vi "Scalar JSON text to Variant.vi"(6 "Type":T1, 8 "error in (no error)":errorcluster, 9 "Variant (Data Type)":variant, 10 "Offset":i32, 11 "JSON":string) -> (0 "error out":errorcluster, 1 "Variant out":variant)   [LabVIEW 2017, in "JSONtext.lvlib"]
uses:
  JSONtext.lvlib
  <vilib>/Utility/Data Type/Type Definitions/Data Type.ctl
  <vilib>/Utility/Data Type/Type Definitions/Refnum Type.ctl
  Advance past String.vi
  String Subset.vi
  support/Strip Quotes and Unescape.vi
  support/Get Number Text.vi
  NaN or null to Integer ERROR.vi
  Advance past Number.vi
  Parsing Error in converting to LabVIEW type.vi
  support/Unescape JSON string.vi
  <vilib>/JDP Science/JDP Science Common Utilities/Timestamp/Text to Timestamp.vi
  <vilib>/Utility/Data Type/NI_Data Type.lvlib
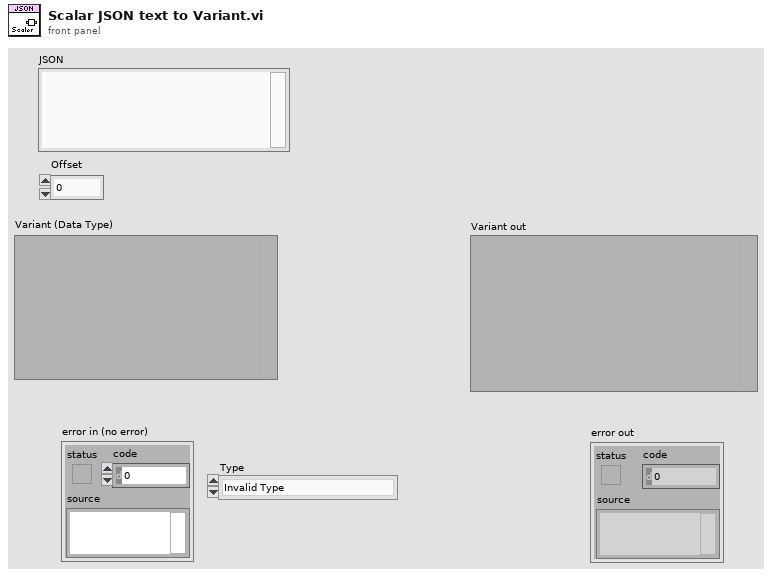
[diagram p1: front panel]
types:
  T1 = typedef "NI_Data Type.lvlib/Data Type.ctl" = enum8{"Invalid Type", "Void", "I8", "I16", "I32", "I64", "U8", "U16", "U32", "U64", "Single Float", "Double Float", "Extended Float", "Single Complex", "Double Complex", "Extended Complex", "Enum U8", "Enum U16", "Enum U32", "Enum U64", "Single Float With Unit", "Double Float With Unit", "Extended Float With Unit", "Single Complex with Unit", "Double Complex with Unit", "Extended Complex with Unit", "Boolean", "String", "Path", "Picture", "Tag", "Array", "Cluster", "Variant", "LV Variant", "Waveform", "Timestamp", "Digital Waveform", "Digital Data", "ExpressData", "Refnum", "External Data", "VI", "Poly VI", "LabVIEW Class Instance", "Fixed Point"}
  T2 = typedef "JSONtext.lvlib/Parsing State.ctl" = enum16{"Parser Error", "Object", "Array", "String", "Number/Other", "Leading Whitespace", "Object end", "Array end", "Value end"}
  T3 = typedef "NI_Data Type.lvlib/Refnum Type.ctl" = enum16{"NotARefnum", "UnknownRefnum", "Generic", "Datalog", "ByteStream", "Device", "Occurence", "TCPNetConnection", "Auto", "Menu", "Imaq", "Hardware", "DataSocket", "Visa", "IVI", "UDPNetConnection", "Notifier", "Queue", "Irda", "EventReg", "DotNet", "UserEvent", "Callback", "UNUSED_EMPTY_POSITION", "BlueToothNetConnection", "LVObjApp", "LVObjVI", "LVObjUnknown", "GenericClass", "UserDefinedRefnumTag", "DataValue", "RT FIFO", "TDMS File"}
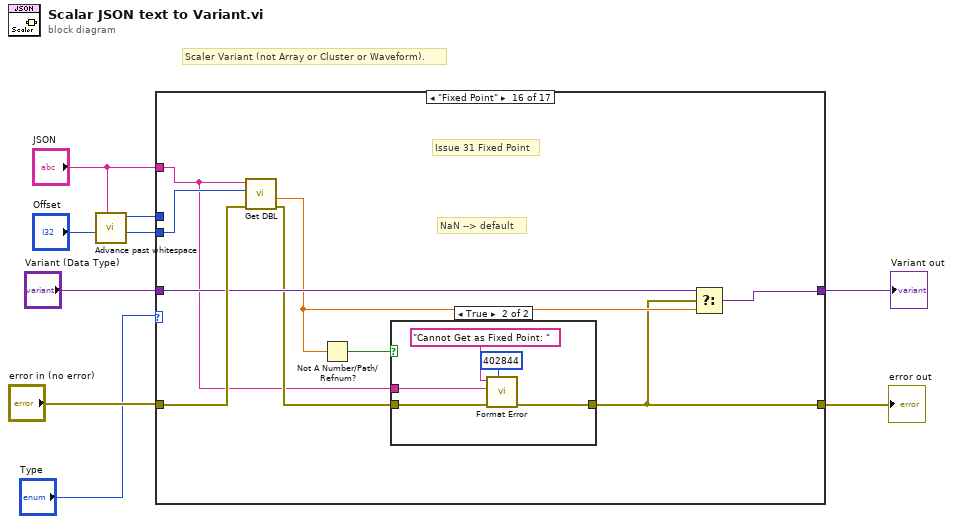
[diagram p0: block diagram]
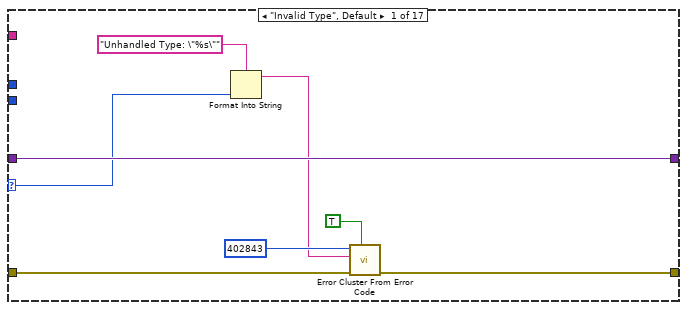
[diagram p2: hidden frame]
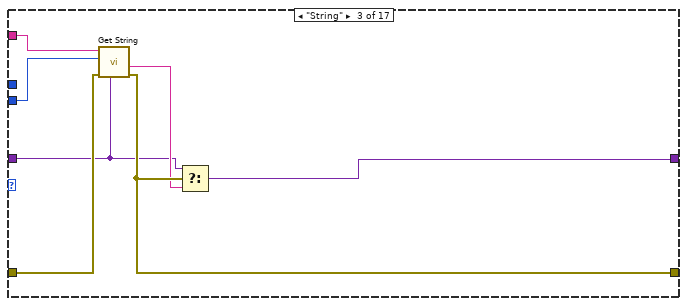
[diagram p4: hidden frame]
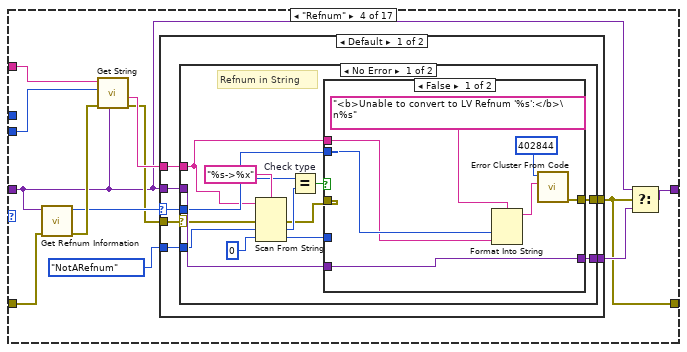
[diagram p5: hidden frame]
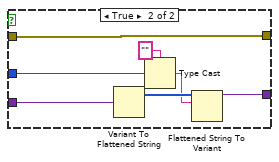
[diagram p6: hidden frame]
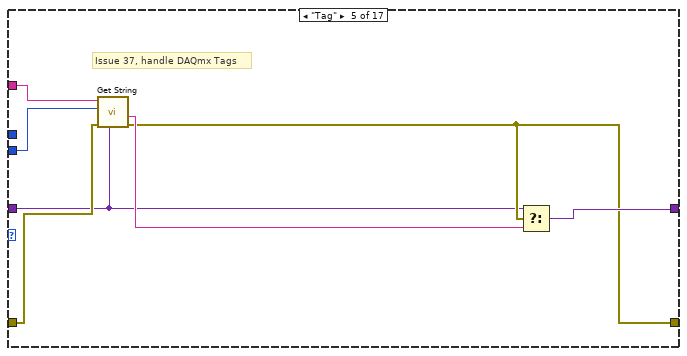
[diagram p9: hidden frame]
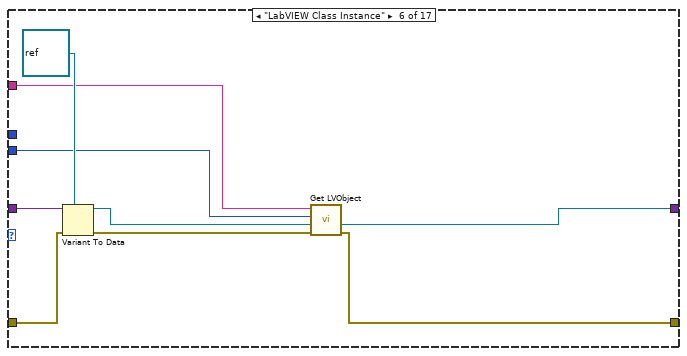
[diagram p10: hidden frame]
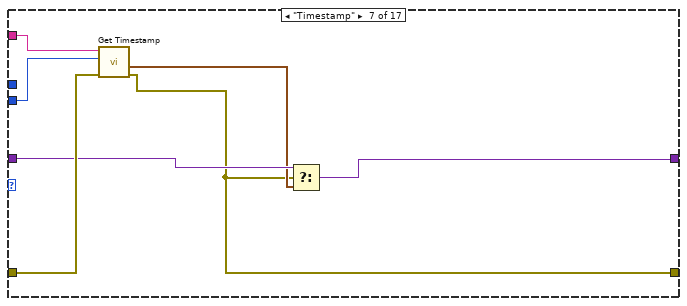
[diagram p11: hidden frame]
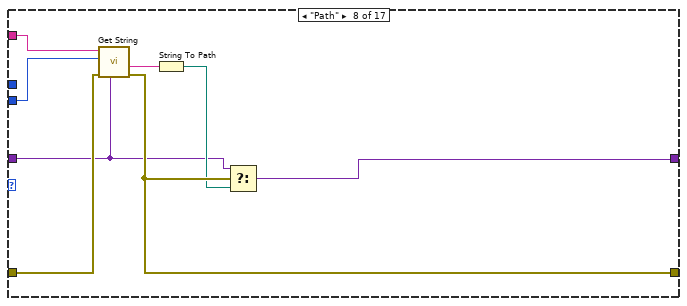
[diagram p12: hidden frame]
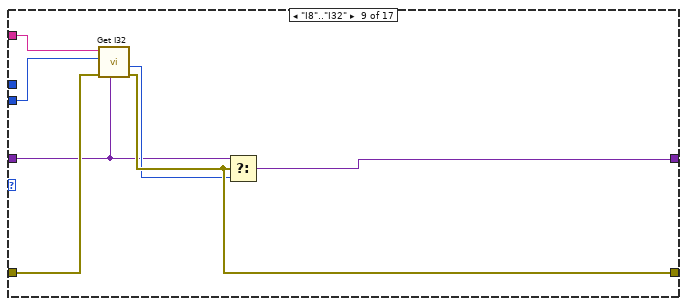
[diagram p13: hidden frame]
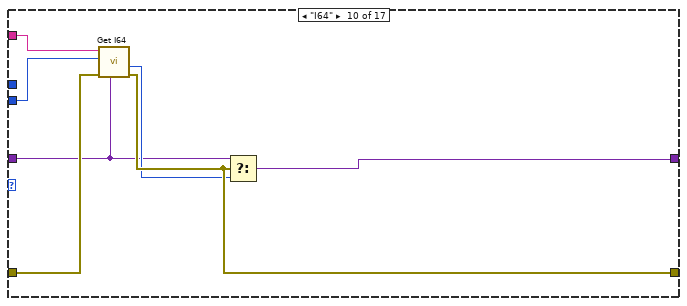
[diagram p14: hidden frame]
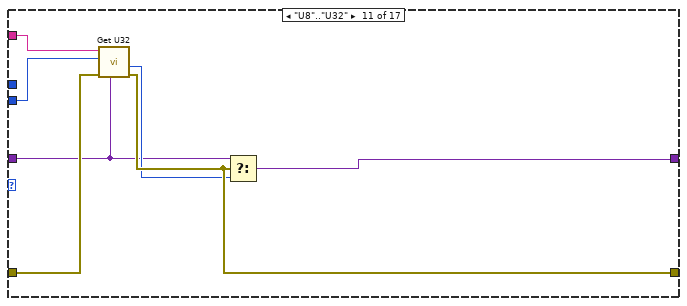
[diagram p15: hidden frame]
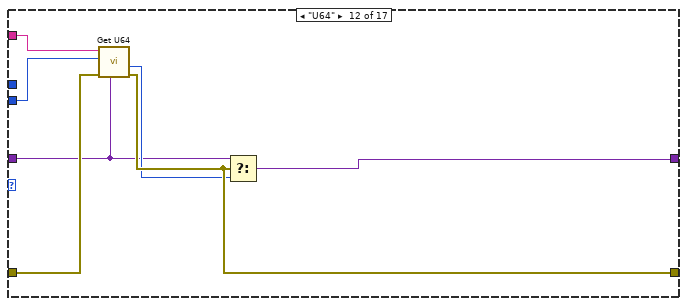
[diagram p16: hidden frame]
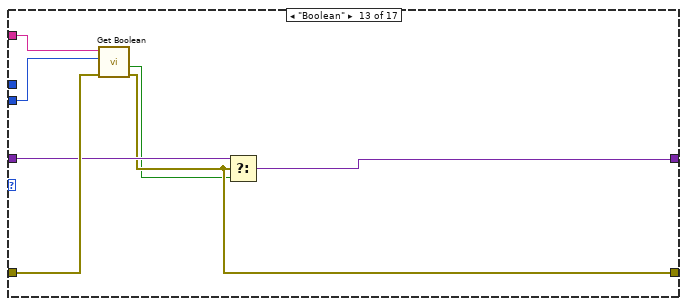
[diagram p17: hidden frame]
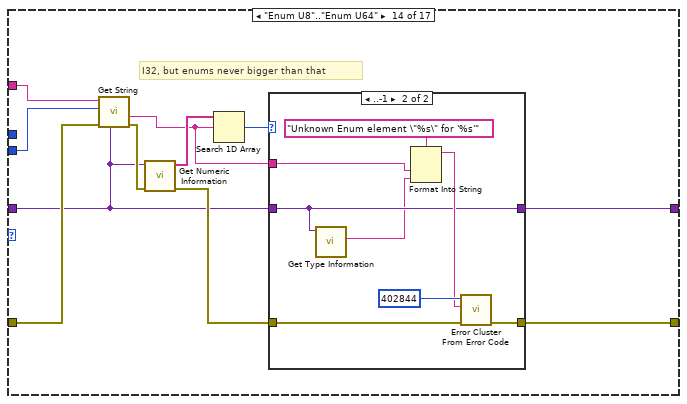
[diagram p18: hidden frame]
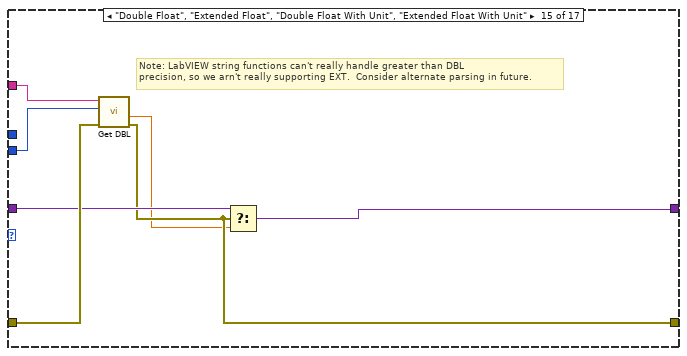
[diagram p20: hidden frame]
diagram:
  # "Scaler Variant (not Array or Cluster or Waveform)."
  n1 = call "Advance past whitespace.vi"("JSON"="JSON", "Offset"="Offset") -> ("Offset of first non-whitespace"=w5:i32, "Parser State"=w3:T2)  [unwired: 8 in]
  n2 = case shown="\"Fixed Point\"" "Type" {
    selector: "Type" -> [w12 _ _ _ _ _ _ _ _ _ _ _ _ _ _ _ _]
    tunnel: "Variant (Data Type)" -> [w16 w18 w20 w27 w76 w90 w95 w99 w107 w114 w121 w128 w139 w142 w167 w176 w189]
    tunnel: "JSON" -> [_ _ w25 w37 w81 w84 w97 w105 w109 w116 w123 w130 w136 w150 w164 w172 w186]
    tunnel: [w15 w19 w22 w29 w77 w89 w92 w102 w110 w117 w124 w131 w137 w146 w165 w170 w187] -> w8
    tunnel: "error in (no error)" -> [w17 w19 w24 w35 w79 w88 w96 w104 w112 w119 w126 w133 w140 w151 w168 w177 w190]
    tunnel: w5 -> [_ _ w26 w38 w82 w85 w98 w106 w113 w120 w127 w134 w141 w152 w169 w178 w191]
    tunnel: [w16 w18 w23 w36 w80 w83 w94 w103 w111 w118 w125 w132 w138 w147 w166 w175 w188] -> w7
    tunnel: w3 -> [_ _ _ _ _ _ _ _ _ _ _ _ _ _ _ _ _]
    frame "Invalid Type", Default {
      n3 = Format Into String(format string="Unhandled Type: \"%s\"", w12) -> (resulting string=w10:string)  [unwired: 2 in, 1 out]
      n4 = call <vilib>:"Error Cluster From Error Code.vi"("show call chain? (False)"=TRUE, "error in (no error)"=w17, "error message (\"\")"=w10, "error code (0)"=402843) -> ("error out"=w15:errorcluster)  [unwired: 5 in]
    }
    frame "Void" {
      # "Empty Variant: #ToDo Variant Attributes?"
    }
    frame "String" {
      n5 = call "Get String.vi"("LV Type"=w20, "error in (no error)"=w24, "Offset"=w26, "JSON"=w25) -> ("error out"=w22:errorcluster, "String"=w21:string)  [unwired: 5 in, 1 out]
      n6 = Select(t=w20, s=w22, f=w21) -> (s? t:f=w23:variant)
    }
    frame "Refnum" {
      n7 = call <vilib>:"Get Refnum Information.vi"("error in (no error)"=w35, "Variant"=w27) -> ("error out"=w34:errorcluster, "Reference Type"=w33:T3)  [unwired: 6 in, 2 out]
      n8 = call "Get String.vi"("LV Type"=w27, "error in (no error)"=w34, "Offset"=w38, "JSON"=w37) -> ("error out"=w30:errorcluster, "String"=w31:string)  [unwired: 5 in, 1 out]
      n9 = case shown="Default" w33 {
        selector: w33 -> [w39 _]
        tunnel: [w44 w75] -> w32
        tunnel: w31 -> [w41 w75]
        tunnel: w27 -> [w45 _]
        tunnel: w30 -> [w43 w74]
        tunnel: [w42 w74] -> w29
        tunnel: Refnum_Type."NotARefnum" ("Reference Type") -> [w40 _]
        frame Default {
          n10 = case shown="No Error" w43 {
            selector: w43 -> [w53 w73]
            tunnel: w45 -> [w58 _]
            tunnel: [w57 _] -> w44
            tunnel: [w48 w73] -> w42
            tunnel: w41 -> [w46 _]
            tunnel: w40 -> [w52 _]
            tunnel: w39 -> [w47 _]
            frame No Error {
              # "Refnum in String"
              n11 = Scan From String(format string="%s->%x", input string=w46, error in=w53, default 1=w52, default 2=u32 0) -> (error out=w49:errorcluster, output 1=w51:T3, output 2=w54:u32)  [unwired: 1 in, 2 out]
              n12 = Equal? "Check type"(x=w47, y=w51) -> (x = y?=w50:bool)
              n13 = case shown="False" w50 {
                tunnel: w58 -> [w65 w70]
                tunnel: [w65 w69] -> w57
                tunnel: w54 -> [_ w67]
                tunnel: w49 -> [_ w66]
                tunnel: [w64 w66] -> w48
                tunnel: w47 -> [w60 _]
                tunnel: w46 -> [w59 _]
                frame False {
                  n14 = Format Into String(format string="<b>Unable to convert to LV Refnum '%s':</b>\n%s", w60, w59) -> (resulting string=w62:string)  [unwired: 2 in, 1 out]
                  n15 = call "Error Cluster From Code.vi"("error message (\"\")"=w62, "error code (402840+)"=402844) -> ("error out"=w64:errorcluster)  [unwired: 7 in]
                }
                frame True {
                  n16 = Variant To Flattened String(Variant=w70) -> (1:w72:i16[])  [unwired: 1 out]
                  n17 = Type Cast(type="", x=w67) -> (*(type *) &x=w71:string)
                  n18 = Flattened String To Variant(6:w71, 7:w72) -> (3:w69:variant)  [unwired: 1 in, 1 out]
                }
              }
            }
            frame Error {
            }
          }
        }
        frame "Visa", "IVI", "UserDefinedRefnumTag" {
        }
      }
      n19 = Select(t=w27, s=w29, f=w32) -> (s? t:f=w36:variant)
    }
    frame "Tag" {
      # "Issue 37, handle DAQmx Tags"
      n20 = call "Get String.vi"("LV Type"=w76, "error in (no error)"=w79, "Offset"=w82, "JSON"=w81) -> ("error out"=w77:errorcluster, "String"=w78:string)  [unwired: 5 in, 1 out]
      n21 = Select(t=w76, s=w77, f=w78) -> (s? t:f=w80:variant)
    }
    frame "LabVIEW Class Instance" {
      n22 = Variant To Data(error in=w88, type=refnum<class> refnum ("LabVIEW Object"), Variant=w90) -> (data=w86:refnum<class>, error out=w87:errorcluster)
      n23 = call "Get LVObject.vi"("error in (no error)"=w87, "Object Type"=w86, "Offset"=w85, "JSON String containing Flattened Object"=w84) -> ("error out"=w89:errorcluster, "Object out"=w83:refnum<class>)  [unwired: 5 in, 1 out]
    }
    frame "Timestamp" {
      n24 = call "Get Timestamp.vi"("error in (no error)"=w96, "Offset"=w98, "JSON"=w97) -> ("error out"=w92:errorcluster, "Timestamp"=w93:timestamp)  [unwired: 6 in, 1 out]
      n25 = Select(t=w95, s=w92, f=w93) -> (s? t:f=w94:variant)
    }
    frame "Path" {
      n26 = call "Get String.vi"("LV Type"=w99, "error in (no error)"=w104, "Offset"=w106, "JSON"=w105) -> ("error out"=w102:errorcluster, "String"=w100:string)  [unwired: 5 in, 1 out]
      n27 = String To Path(string=w100) -> (path=w101:path)
      n28 = Select(t=w99, s=w102, f=w101) -> (s? t:f=w103:variant)
    }
    frame "I8".."I32" {
      n29 = call "Get I32.vi"("LV Type"=w107, "error in (no error)"=w112, "Offset"=w113, "JSON"=w109) -> ("error out"=w110:errorcluster, "Number"=w108:i32)  [unwired: 5 in, 1 out]
      n30 = Select(t=w107, s=w110, f=w108) -> (s? t:f=w111:variant)
    }
    frame "I64" {
      n31 = call "Get I64.vi"("LV Type"=w114, "error in (no error)"=w119, "Offset"=w120, "JSON"=w116) -> ("error out"=w117:errorcluster, "Number"=w115:i64)  [unwired: 5 in, 1 out]
      n32 = Select(t=w114, s=w117, f=w115) -> (s? t:f=w118:variant)
    }
    frame "U8".."U32" {
      n33 = call "Get U32.vi"("LV Type"=w121, "error in (no error)"=w126, "Offset"=w127, "JSON"=w123) -> ("error out"=w124:errorcluster, "Number"=w122:u32)  [unwired: 5 in, 1 out]
      n34 = Select(t=w121, s=w124, f=w122) -> (s? t:f=w125:variant)
    }
    frame "U64" {
      n35 = call "Get U64.vi"("LV Type"=w128, "error in (no error)"=w133, "Offset"=w134, "JSON"=w130) -> ("error out"=w131:errorcluster, "Number"=w129:u64)  [unwired: 5 in, 1 out]
      n36 = Select(t=w128, s=w131, f=w129) -> (s? t:f=w132:variant)
    }
    frame "Boolean" {
      n37 = call "Get Boolean.vi"("error in (no error)"=w140, "Offset"=w141, "JSON"=w136) -> ("error out"=w137:errorcluster, "Boolean"=w135:bool)  [unwired: 6 in, 1 out]
      n38 = Select(t=w139, s=w137, f=w135) -> (s? t:f=w138:variant)
    }
    frame "Enum U8".."Enum U64" {
      # "I32, but enums never bigger than that"
      n39 = call "Get String.vi"("LV Type"=w142, "error in (no error)"=w151, "Offset"=w152, "JSON"=w150) -> ("error out"=w144:errorcluster, "String"=w145:string)  [unwired: 5 in, 1 out]
      n40 = call <vilib>:"Get Numeric Information.vi"("error in (no error)"=w144, "Variant"=w142) -> ("error out"=w143:errorcluster, "Enum Names"=w148:string[])  [unwired: 6 in, 2 out]
      n41 = Search 1D Array(1D array=w148, element=w145) -> (index of element=w149:i32)  [unwired: 1 in]
      n42 = case shown="..-1" w149 {
        selector: w149 -> [w153 _]
        tunnel: [w153 w157] -> w147
        tunnel: w142 -> [_ w157]
        tunnel: w143 -> [w154 w160]
        tunnel: [w154 w162] -> w146
        tunnel: w145 -> [_ w155]
        frame 0.. {
        }
        frame ..-1 {
          n43 = call <vilib>:"Get Type Information.vi"("Variant"=w157) -> ("Name"=w156:string)  [unwired: 6 in, 4 out]
          n44 = Format Into String(format string="Unknown Enum element \"%s\" for '%s'", w155, w156) -> (resulting string=w158:string)  [unwired: 2 in, 1 out]
          n45 = call <vilib>:"Error Cluster From Error Code.vi"("error in (no error)"=w160, "error message (\"\")"=w158, "error code (0)"=402844) -> ("error out"=w162:errorcluster)  [unwired: 6 in]
        }
      }
    }
    frame "Double Float", "Extended Float", "Double Float With Unit", "Extended Float With Unit" {
      # "Note: LabVIEW string functions can't really handle greater than DBL\nprecision, so we arn't really supporting EXT.  Consider alternate parsing in future."
      n46 = call "Get DBL.vi"("error in (no error)"=w168, "Offset"=w169, "JSON"=w164) -> ("error out"=w165:errorcluster, "Number"=w163:dbl)  [unwired: 6 in, 1 out]
      n47 = Select(t=w167, s=w165, f=w163) -> (s? t:f=w166:variant)
    }
    frame "Fixed Point" {
      # "NaN --> default"
      # "Issue 31 Fixed Point"
      n48 = call "Get DBL.vi"("error in (no error)"=w177, "Offset"=w178, "JSON"=w172) -> ("error out"=w173:errorcluster, "Number"=w174:dbl)  [unwired: 6 in, 1 out]
      n49 = Not A Number/Path/Refnum?(number/path/refnum=w174) -> (NaN/Path/Refnum?=w171:bool)
      n50 = case shown="True" w171 {
        tunnel: w173 -> [w179 w184]
        tunnel: [w179 w183] -> w170
        tunnel: w172 -> [_ w180]
        frame False {
        }
        frame True {
          n51 = call "Format Error.vi"("error code (402842)"=402844, "error in (no error)"=w184, "message part 2"=w180, "error message"="Cannot Get as Fixed Point: " ("format string")) -> ("error out"=w183:errorcluster)  [unwired: 7 in]
        }
      }
      n52 = Select(t=w176, s=w170, f=w174) -> (s? t:f=w175:variant)
    }
    frame "Single Float", "Single Float With Unit" {
      n53 = call "Get SGL.vi"("error in (no error)"=w190, "Offset"=w191, "JSON"=w186) -> ("error out"=w187:errorcluster, "Number"=w185:sgl)  [unwired: 6 in, 1 out]
      n54 = Select(t=w189, s=w187, f=w185) -> (s? t:f=w188:variant)
    }
  }
  "Variant out" <- w7
  "error out" <- w8
